vi "CalculateAccuracy.vi"(9 "metrics":T1, 10 "Number of tries":refnum<vi>, 11 "Correct interpretations":refnum<vi>) -> (3 "Accuracy":dbl)   [LabVIEW 2017, in "LeapMotion.lvlib"]
uses:
  LeapMotion.lvlib
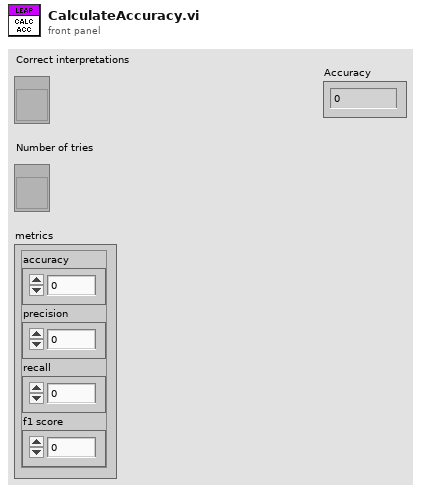
[diagram p1: front panel]
types:
  T1 = cluster{"accuracy":dbl, "precision":dbl, "recall":dbl, "f1 score":dbl}
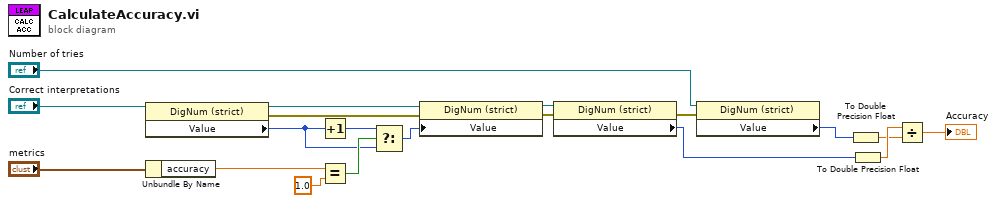
[diagram p0: block diagram]
diagram:
  n1 = property class="DigNum (strict)"(reference="Correct interpretations") -> (reference out=w2:refnum<vi>, error out=w11:errorcluster, "Value"=w1:i32)  [unwired: 1 in]
  n2 = Unbundle By Name("metrics") -> ("accuracy"=w14:dbl)
  n3 = Increment(x=w1) -> (x+1=w18:i32)
  n4 = Equal?(x=w14, y=1.0) -> (x = y?=w16:bool)
  n5 = Select(t=w18, s=w16, f=w1) -> (s? t:f=w17:i32)
  n6 = property class="DigNum (strict)"(reference=w2, error in=w11, "Value"=w17) -> (reference out=w9:refnum<vi>, error out=w10:errorcluster)
  n7 = property class="DigNum (strict)"(reference=w9, error in=w10) -> (error out=w8:errorcluster, "Value"=w6:i32)  [unwired: 1 out]
  n8 = property class="DigNum (strict)"(reference="Number of tries", error in=w8) -> ("Value"=w7:i32)  [unwired: 2 out]
  n9 = To Double Precision Float(number=w7) -> (double precision float=w4:dbl)
  n10 = To Double Precision Float(number=w6) -> (double precision float=w5:dbl)
  n11 = Divide(x=w5, y=w4) -> (x/y=→"Accuracy":dbl)
